vi "decimal string to hex string.vi"(10 "Decimal String":string) -> (2 "Hex String":string)   [LabVIEW 8.6]
doc: "This VI convert decimal string to raw hex string."
panel:
  # "decimal string to hex string.vi\nConvert decimal string to raw hex string.\n\ncaozijian.cn@gmail.com"
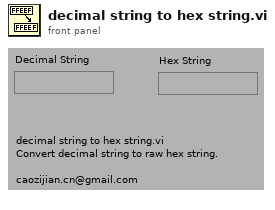
[diagram p1: front panel]
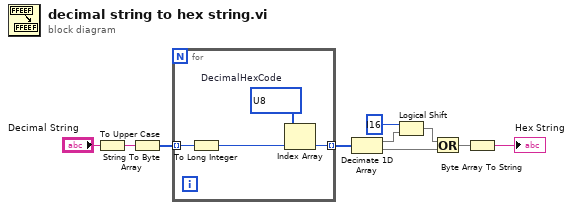
[diagram p0: block diagram]
diagram:
  n1 = To Upper Case(1:"Decimal String") -> (0:w3:string)
  n2 = String To Byte Array(string=w3) -> (unsigned byte array=w10:u8[])
  n3 = for {
    tunnel: w10 -> [w13] mode=indexing
    tunnel: [w12] -> w9 mode=indexing
    w14 = u8[] ?  # DecimalHexCode
    n4 = To Long Integer(number=w13) -> (32bit integer=w11:i32)
    n5 = Index Array(array=w14, index=w11) -> (element=w12:u8)
  }
  n6 = Decimate 1D Array(w9) -> (w8:u8[], w5:u8[])
  n7 = Logical Shift(y=i16 ?, x=w8) -> (x << y=w6:u8[])
  n8 = Or(x=w6, y=w5) -> (x .or. y?=w4:u8[])
  n9 = Byte Array To String(unsigned byte array=w4) -> (string=→"Hex String":string)
